vi "ViewObject.vi"(6 "y":bool, 8 "error in":errorcluster, 10 "New Image":T1) -> (0 "error out":errorcluster, 2 "Image Out fgv":T1(plugin-control), 3 "Number of Particles (Particle Analysis 1)":i32)   [LabVIEW 2019]
uses:
  <vilib>/vision/Image Controls.llb/IMAQ Image.ctl
  KNRm_ReMi_OS6_64Motor.lvlibp
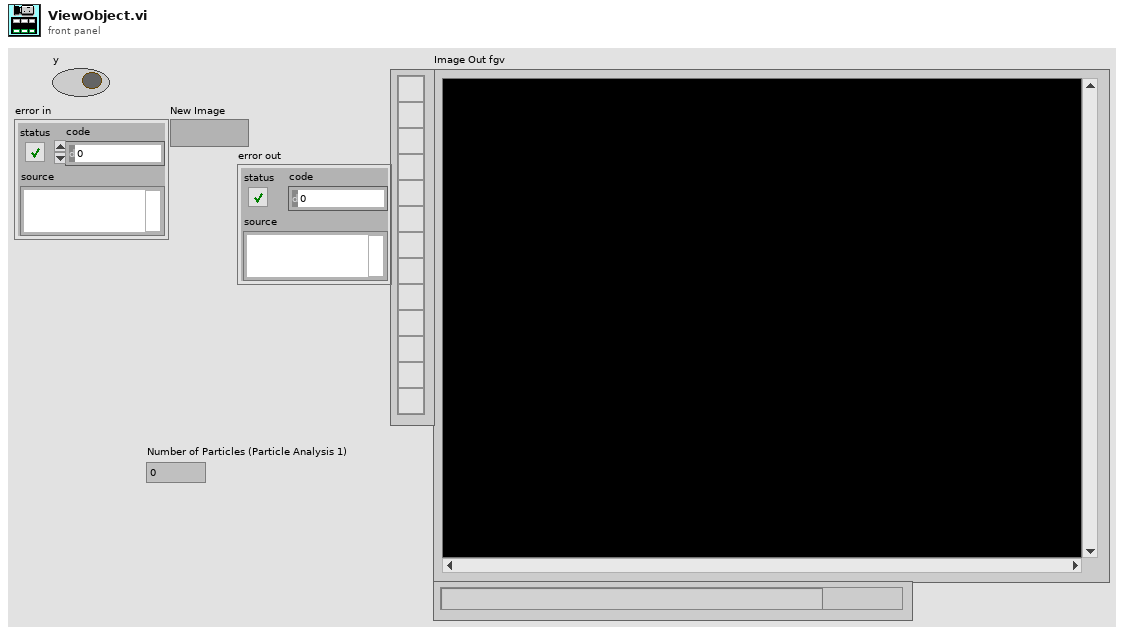
[diagram p1: front panel]
types:
  T1 = typedef "IMAQ Image.ctl" = refnum<image>
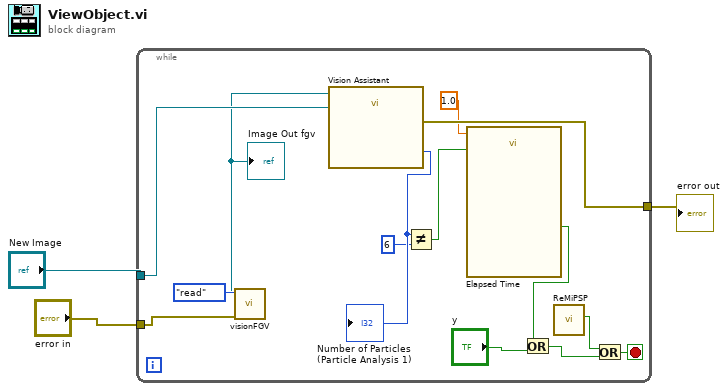
[diagram p0: block diagram]
diagram:
  n1 = while {
    tunnel: "error in" -> [w16]
    tunnel: "New Image" -> [w15]
    tunnel: [w12] -> w1
    stop <- w4 stop-if-true
    n2 = call "visionFGV.vi"("Error In"=w16, "Function"=enum16{"set", "read", "close"}."read") -> ("Image Out fgv"=w14:T1)  [unwired: 8 in, 1 out]
    "Image Out fgv" <- w14
    n3 = call "Vision Assistant"("Image In"=w14, "Image Dst"=w15) -> ("Number of Particles (Particle Analysis 1)"=w11:i32, "error out"=w12:errorcluster)  [unwired: 23 in, 1 out]
    "Number of Particles (Particle Analysis 1)" <- w11
    n4 = Not Equal?(x=w11, y=6) -> (x != y?=w9:bool)
    n5 = call "Elapsed Time"("Time Target (s)"=1.0, "Reset"=w9) -> ("Time has Elapsed"=w7:bool)  [unwired: 10 in, 7 out]
    n6 = Or(x=w7, y="y") -> (x .or. y?=w6:bool)
    n7 = call "ReMiPSP.vi"() -> ("EMS"=w5:bool)  [unwired: 9 in, 2 out]
    n8 = Or(x=w5, y=w6) -> (x .or. y?=w4:bool)
  }
  "error out" <- w1
